vi "DialogCloneMethod.vi"(0 "ClassWriter.lvclass":refnum<class "ClassWriter.lvclass">, 1 "VIItemRefIn":refnum<vi>, 5 "error in (no error)":errorcluster) -> (11 "NewVIDescriptionOut":string caption="New VI Description", 13 "OpenAfter":bool, 14 "ClassWriter.lvclassOut":refnum<class "ClassWriter.lvclass">, 15 "VIItemRefOut":refnum<vi>, 16 "NewVIPath":path, 17 "Cancelled":bool, 18 "LibraryOwners":refnum<vi>[](array[refnum]), 19 "error out":errorcluster)   [LabVIEW 2020, in "ClassWriter.lvclass"]
uses:
  <resource>/Framework/Providers/Open_GDS/ClassProviders/Provider_BaseClassInterface/ClassWriter_class/ClassWriter.lvclass
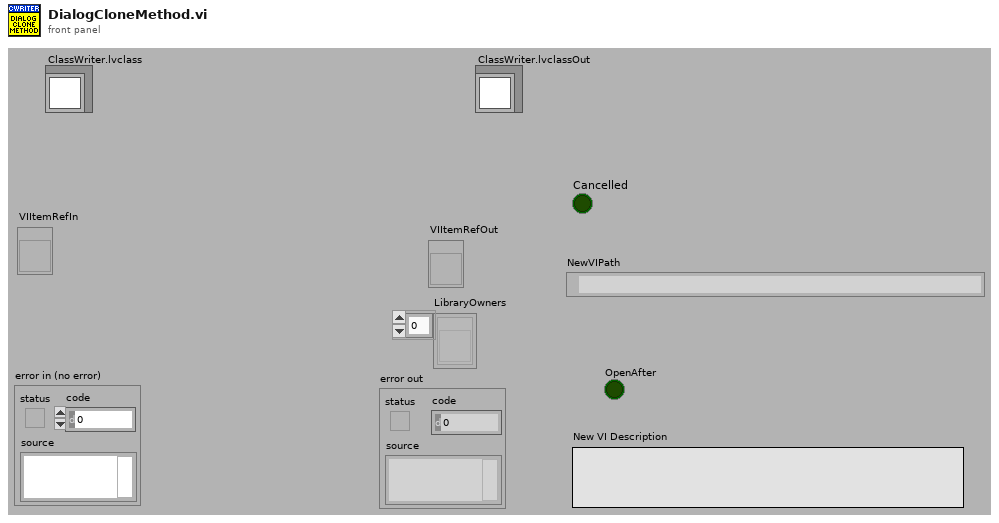
[diagram p1: front panel]
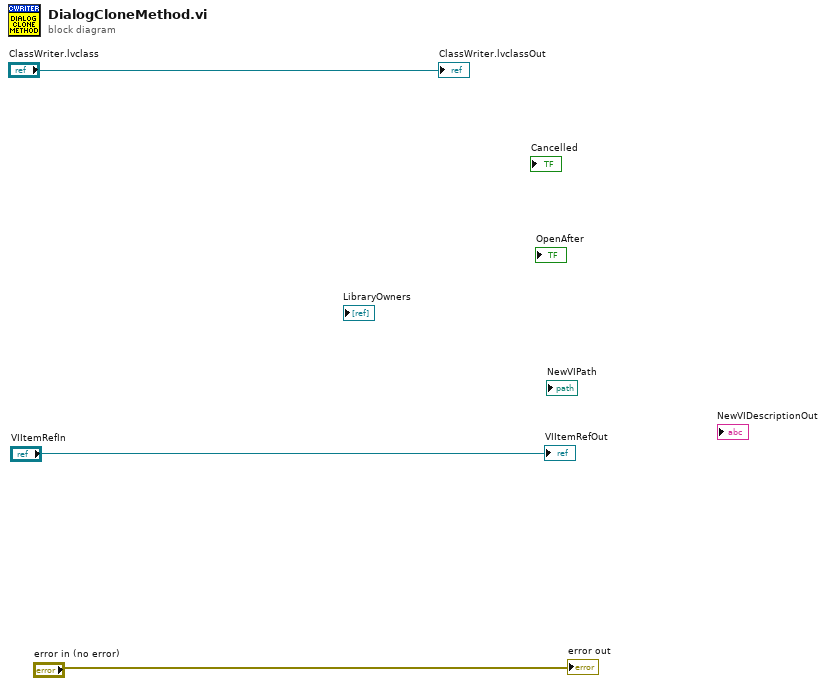
[diagram p0: block diagram]
diagram:
  "VIItemRefOut" <- "VIItemRefIn"
  "error out" <- "error in (no error)"
  "ClassWriter.lvclassOut" <- "ClassWriter.lvclass"
